vi "SUB_EnergyToChannel.vi"(1 "Intercept":dbl, 2 "Slope":dbl, 3 "Energy":dbl) -> (0 "Channel":u32)   [LabVIEW 2015]
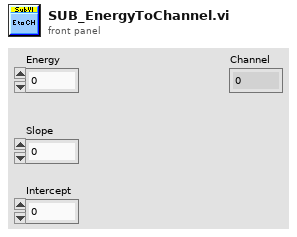
[diagram p1: front panel]
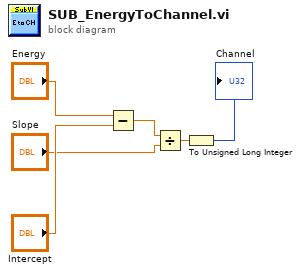
[diagram p0: block diagram]
diagram:
  n1 = Subtract(x="Energy", y="Intercept") -> (x-y=w4:dbl)
  n2 = Divide(x=w4, y="Slope") -> (x/y=w2:dbl)
  n3 = To Unsigned Long Integer(number=w2) -> (unsigned 32bit integer=→"Channel":u32)
